vi "inverse.vi"(8 "RobotParams":T1={"R1"=31.0, "R2"=37.0, "R3"=31.0, "RadsPerCnt"=0.0, "EncOffset1"=0, "EncOffset2"=0, "HomeX"=0.0, "HomeY"=0.0}, 10 "Y":dbl, 11 "X":dbl) -> (1 "Enc 2":i32, 2 "Enc 1":i32)   [LabVIEW 2019]
uses:
  RobotParams.ctl
  <vilib>/imath/engines/lvmath2/RunTimeEngine/BuiltInFunctions/atan/NIMS_atan(C).vi
  <instcachedir>/0/NIMS_atan(C)_0A85D365582D4E8AB3874BC9125E138E.lvgen/NIMS_atan(C)_0A85D365582D4E8AB3874BC9125E138E_001.vi
  <vilib>/imath/engines/lvmath2/RunTimeEngine/BuiltInFunctions/int32/NIMS_int32(complex).vi
  <instcachedir>/0/NIMS_int32(complex)_4AFAE466A00040C78D20A2691237067B.lvgen/NIMS_int32(complex)_4AFAE466A00040C78D20A2691237067B_001.vi
  <vilib>/imath/engines/lvmath2/RunTimeEngine/NodeEndStatement/NIMS_NodeEndStatement_Output.vi
  <instcachedir>/0/NIMS_NodeEndStatement_Output_53EC0D466D134D7ABD903AC30B43404B.lvgen/NIMS_NodeEndStatement_Output_53EC0D466D134D7ABD903AC30B43404B_009.vi
  <vilib>/imath/engines/lvmath2/RunTimeEngine/ErrorHandling/NIMS_Finalize Error.vi
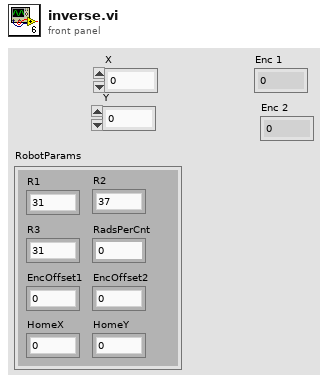
[diagram p1: front panel]
types:
  T1 = typedef "RobotParams.ctl" = cluster{"R1":dbl, "R2":dbl, "R3":dbl, "RadsPerCnt":dbl, "EncOffset1":i32, "EncOffset2":i32, "HomeX":dbl, "HomeY":dbl}
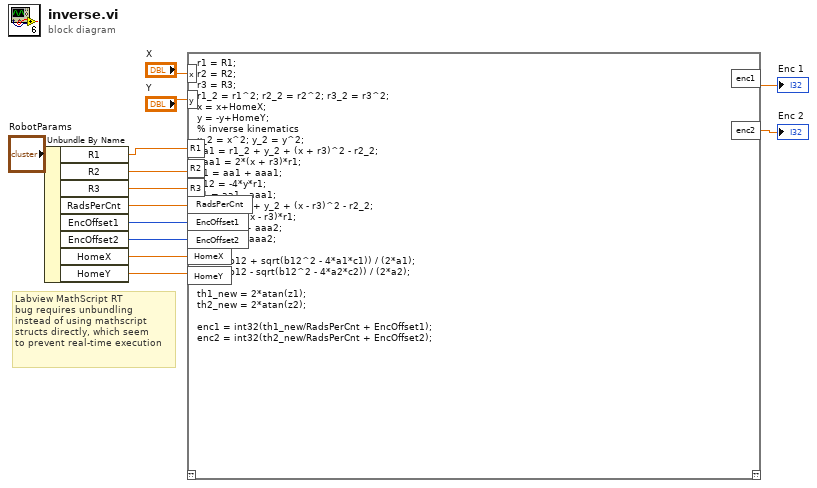
[diagram p0: block diagram]
diagram:
  # "Labview MathScript RT\nbug requires unbundling\ninstead of using mathscript\nstructs directly, which seem\nto prevent real-time execution"
  n1 = Unbundle By Name("RobotParams") -> ("R1"=w8:dbl, "R2"=w7:dbl, "R3"=w6:dbl, "RadsPerCnt"=w5:dbl, "EncOffset1"=w4:i32, "EncOffset2"=w3:i32, "HomeX"=w2:dbl, "HomeY"=w1:dbl)
  n2 = mathscript code="r1 = R1;\nr2 = R2;\nr3 = R3;\nr1_2 = r1^2; r2_2 = r2^2; r3_2 = r3^2;\nx = x+HomeX;\ny = -y+HomeY;\n% inverse kinematics\nx_2 = x^2; y_2 = y^2;\naa1 = r1_2 + y_2 + (x + r3)^2 - r2_2;\naaa1 = 2*(x + r3)*r1;\na1 = aa1 + aaa1;\nb12 = -4*y*r1;\nc1 = aa1 - aaa1;\naa2 = r1_2 + y_2 + (x - r3)^2 - r2_2;\naaa2 = 2*(x - r3)*r1;\na2 = aa2 + aaa2;\nc2 = aa2 - aaa2;\n\nz1 = (-b12 + sqrt(b12^2 - 4*a1*c1)) / (2*a1);\nz2 = (-b12 - sqrt(b12^2 - 4*a2*c2)) / (2*a2);\n\nth1_new = 2*atan(z1);\nth2_new = 2*atan(z2);\n\nenc1 = int32(th1_new/RadsPerCnt + EncOffset1);\nenc2 = int32(th2_new/RadsPerCnt + EncOffset2);"("x"="X", "y"="Y", "HomeY"=w1, "HomeX"=w2, "EncOffset2"=w3, "EncOffset1"=w4, "RadsPerCnt"=w5, "R3"=w6, "R2"=w7, "R1"=w8) -> ("enc1"=→"Enc 1":cdb, "enc2"=→"Enc 2":cdb)  [unwired: 1 in, 1 out]
